vi "Determine Insert Before Node.vi"(6 "New Node":T1, 8 "error in":errorcluster, 11 "Document in":refnum<k20>) -> (0 "error out":errorcluster, 3 "Document out":refnum<k20>, 4 "Insert Before Node":refnum<k20>)   [LabVIEW 2025]
uses:
  Shared/Types/NodeFilteringOptions.ctl
  Types/New Node Types.ctl
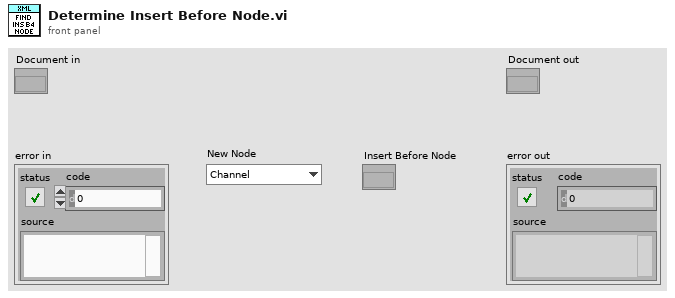
[diagram p1: front panel]
types:
  T1 = typedef "New Node Types.ctl" = enum16{"Channel", "Waveform", "Section"}
  T2 = typedef "NodeFilteringOptions.ctl" = enum16{"GetCustomDeviceNode", "GetAllChannelNodes", "GetAllSectionNodes", "GetAllWaveformNodes", "GetFirstChannelNode", "GetFirstSectionNode", "GetFirstWaveformNode", "GetSpecificSectionNode", "GetSpecificCustomDeviceNode", "GetSpecificChannelNode", "GetSpecificWaveformNode", "GetMatchedNamedNode", "GetEnumDefinitionsNode", "GetSpecificEnumDefinitionNode", "GetAllEnumDefinitionNodes", "GetDynamicChannelNodes"}
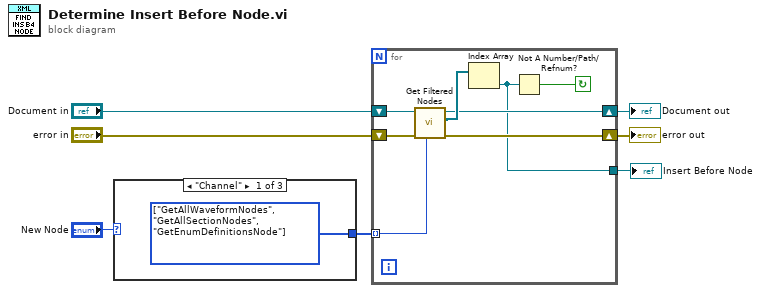
[diagram p0: block diagram]
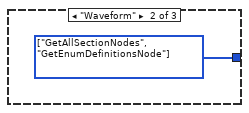
[diagram p2: hidden frame]
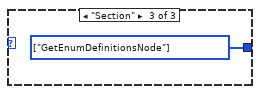
[diagram p3: hidden frame]
diagram:
  n1 = case shown="\"Channel\"" "New Node" {
    tunnel: [w8 w9 w10] -> w4
    frame "Channel" {
      w8 = T2[] [enum."GetAllWaveformNodes", enum."GetAllSectionNodes", enum."GetEnumDefinitionsNode"] items=["GetCustomDeviceNode", "GetAllChannelNodes", "GetAllSectionNodes", "GetAllWaveformNodes", "GetFirstChannelNode", "GetFirstSectionNode", "GetFirstWaveformNode", "GetSpecificSectionNode", "GetSpecificCustomDeviceNode", "GetSpecificChannelNode", "GetSpecificWaveformNode", "GetMatchedNamedNode", "GetEnumDefinitionsNode", "GetSpecificEnumDefinitionNode", "GetAllEnumDefinitionNodes", "GetDynamicChannelNodes"]
    }
    frame "Waveform" {
      w9 = T2[] [enum."GetAllSectionNodes", enum."GetEnumDefinitionsNode"] items=["GetCustomDeviceNode", "GetAllChannelNodes", "GetAllSectionNodes", "GetAllWaveformNodes", "GetFirstChannelNode", "GetFirstSectionNode", "GetFirstWaveformNode", "GetSpecificSectionNode", "GetSpecificCustomDeviceNode", "GetSpecificChannelNode", "GetSpecificWaveformNode", "GetMatchedNamedNode", "GetEnumDefinitionsNode", "GetSpecificEnumDefinitionNode", "GetAllEnumDefinitionNodes", "GetDynamicChannelNodes"]
    }
    frame "Section" {
      w10 = T2[] [enum."GetEnumDefinitionsNode"] items=["GetCustomDeviceNode", "GetAllChannelNodes", "GetAllSectionNodes", "GetAllWaveformNodes", "GetFirstChannelNode", "GetFirstSectionNode", "GetFirstWaveformNode", "GetSpecificSectionNode", "GetSpecificCustomDeviceNode", "GetSpecificChannelNode", "GetSpecificWaveformNode", "GetMatchedNamedNode", "GetEnumDefinitionsNode", "GetSpecificEnumDefinitionNode", "GetAllEnumDefinitionNodes", "GetDynamicChannelNodes"]
    }
  }
  n2 = for {
    tunnel: w4 -> [w16] mode=indexing
    shift-right: [w13] -> w2
    shift-left: "error in" -> [w17]
    shift-right: [w12] -> w3
    shift-left: "Document in" -> [w18]
    tunnel: [w11] -> w1
    stop <- w14 continue-if-true
    n3 = call "Get Filtered Nodes.vi"("Node Filtering"=w16, "error in"=w17, "Document in"=w18) -> ("error out"=w13:errorcluster, "Filtered Nodes"=w15:refnum<k20>[], "Document out"=w12:refnum<k20>)  [unwired: 4 in, 2 out]
    n4 = Index Array(array=w15) -> (element=w11:refnum<k20>)  [unwired: 1 in]
    n5 = Not A Number/Path/Refnum?(number/path/refnum=w11) -> (NaN/Path/Refnum?=w14:bool)
  }
  "Document out" <- w3
  "error out" <- w2
  "Insert Before Node" <- w1
